vi "Decorate.vi"(10 "Event":refnum<class "Event.lvclass">, 11 "TEMPLATE Event in":refnum<class "TEMPLATE Event.lvclass">) -> (3 "TEMPLATE Event out":refnum<class "TEMPLATE Event.lvclass">)   [LabVIEW 2021, in "_Template.lvlib" / "Templates.lvlib" / "TEMPLATE Event.lvlib" / "TEMPLATE Event.lvclass"]
uses:
  TEMPLATE Event.lvclass
  TEMPLATE Event.lvclass/TEMPLATE Event.ctl
  <vilib>/Nathan Davis/jettl/Set Panel State Msg Strategy/Set Panel State Msg Strategy.lvlib
  <vilib>/Nathan Davis/jettl/Setup Msg Strategy/Setup Msg Strategy.lvlib
  <vilib>/Nathan Davis/jettl/jettl/Event/Event.lvclass
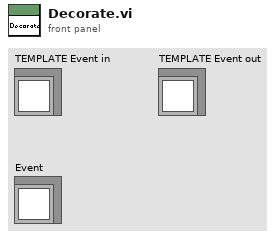
[diagram p1: front panel]
types:
  T1 = enum32{"Invalid", "Standard", "Closed", "Hidden", "Minimized", "Maximized"}
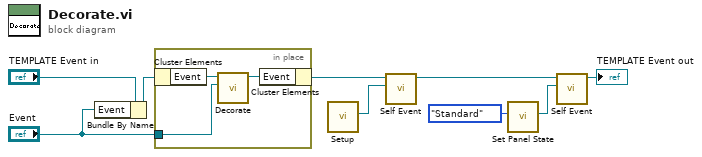
[diagram p0: block diagram]
diagram:
  n1 = Bundle By Name(cluster="TEMPLATE Event in", "Event"="Event") -> (w8:refnum<class "TEMPLATE Event.lvclass">)
  n2 = in-place {
    in-place-border: "Event" -> [w10]
    n3 = in-place-cluster #1(w8) -> ("Event"=w12:refnum<class "Event.lvclass">)
    n4 = call-dynamic "Decorate.vi"("Event"=w10, "Event in"=w12) -> ("Event out"=w11:refnum<class "Event.lvclass">)  [unwired: 9 in]
    n5 = in-place-cluster #1("Event"=w11) -> (w7:refnum<class "TEMPLATE Event.lvclass">)
  }
  n6 = call <vilib>:"Setup.vi"() -> ("Msg Strategy"=w2:refnum<class "Msg Strategy.lvclass">)  [unwired: 11 in]
  n7 = call-dynamic "Self Event.vi"("Msg Strategy"=w2, "TEMPLATE Event in"=w7) -> ("TEMPLATE Event out"=w3:refnum<class "TEMPLATE Event.lvclass">)  [unwired: 9 in]
  n8 = call <vilib>:"Set Panel State.vi"("Front Panel Window:State"=T1."Standard") -> ("Msg Strategy"=w5:refnum<class "Msg Strategy.lvclass">)  [unwired: 10 in]
  n9 = call-dynamic "Self Event.vi"("Msg Strategy"=w5, "TEMPLATE Event in"=w3) -> ("TEMPLATE Event out"=→"TEMPLATE Event out":refnum<class "TEMPLATE Event.lvclass">)  [unwired: 9 in]
